vi "CheckAvailableFsample.vi"() -> ()   [LabVIEW 2022 SP3]
uses:
  <vilib>/Analysis/1siggen.llb/Ramp Pattern by Delta.vi
  <vilib>/DAQmx/configure/timing.llb/DAQmx Timing (Sample Clock).vi
  <resource>/objmgr/daqmx.rc
  <vilib>/Analysis/NI_AALBase.lvlib
  <vilib>/DAQmx/create/channels.llb/DAQmx Create Channel (AI-Voltage-Basic).vi
panel:
  out "error out":errorcluster
  in  "deltaFreq":dbl=1.0 format="%_3pHz"
  in  "minFreq":dbl=1.0 format="%_3pHz"
  in  "maxFreq":dbl=3000.0 format="%_3pHz"
  out "Fcheck":dbl
  out "XY Graph":cluster{dbl[], dbl[]}[](graph)
  in  "physical channels":tag
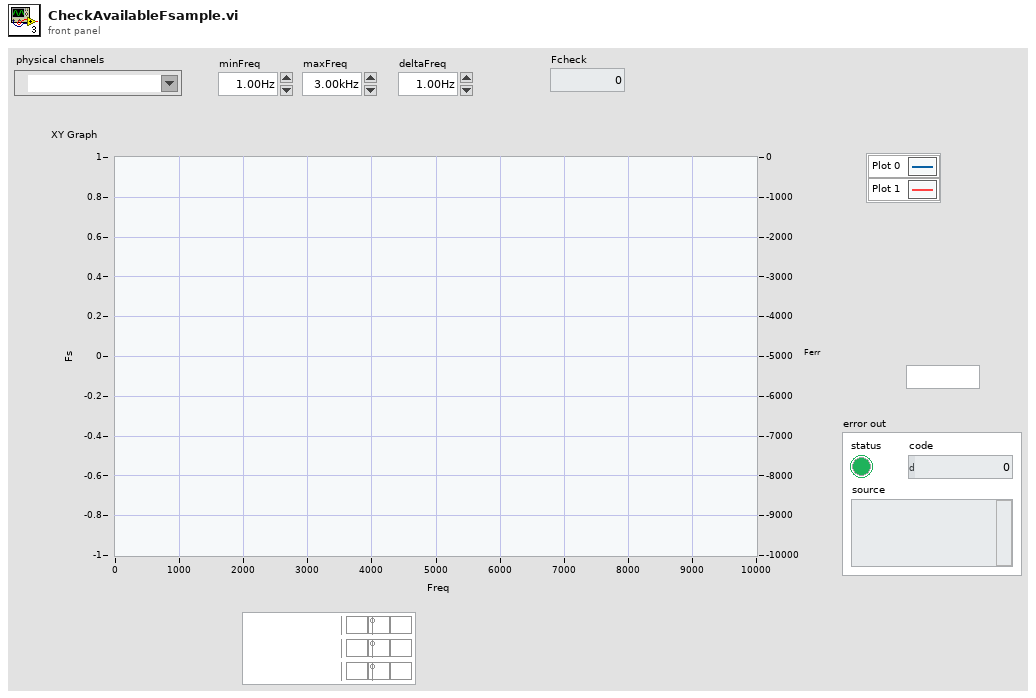
[diagram p1: front panel]
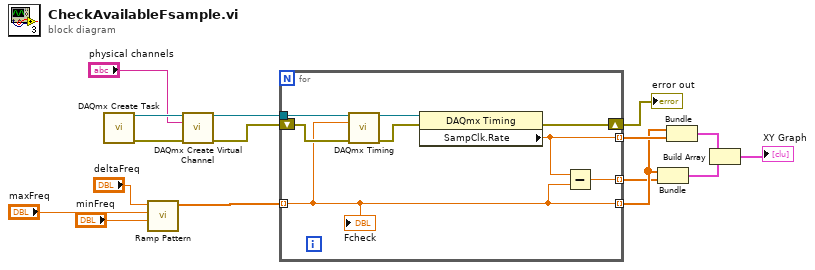
[diagram p0: block diagram]
diagram:
  n1 = call <vilib>:"DAQmx Create Task.vi"() -> ("task out"=w14:refnum<k21>, "error out"=w15:errorcluster)  [unwired: 14 in]
  n2 = call-poly <vilib>:"Ramp Pattern.vi"("start"="minFreq", "end"="maxFreq", "delta"="deltaFreq") -> ("Ramp Pattern"=w8:dbl[])  [unwired: 6 in, 2 out]
  n3 = call-poly <vilib>:"DAQmx Create Virtual Channel.vi"("task in"=w14, "physical channels"="physical channels", "error in"=w15) -> ("task out"=w13:refnum<k21>, "error out"=w16:errorcluster)  [unwired: 11 in]
  n4 = for {
    tunnel: w13 -> [w21]
    tunnel: w8 -> [w20] mode=indexing
    tunnel: [w19] -> w7 mode=indexing
    tunnel: [w20] -> w6 mode=indexing
    tunnel: [w18] -> w5 mode=indexing
    shift-right: [w17] -> w1
    shift-left: w16 -> [w22]
    n5 = call-poly <vilib>:"DAQmx Timing.vi"("task/channels in"=w21, "rate"=w20, "error in"=w22) -> ("task out"=w24:refnum<k21>, "error out"=w23:errorcluster)  [unwired: 4 in, 7 out]
    n6 = property class="DAQmx Timing"(reference=w24, error in=w23) -> (error out=w17:errorcluster, "SampClk.Rate"=w19:dbl)  [unwired: 1 out]
    n7 = Subtract(x=w19, y=w20) -> (x-y=w18:dbl)
    "Fcheck" <- w20
  }
  "error out" <- w1
  n8 = Bundle(w6, w5) -> (w3:cluster{dbl[], dbl[]})  [unwired: 1 in]
  n9 = Bundle(w6, w7) -> (w4:cluster{dbl[], dbl[]})  [unwired: 1 in]
  n10 = Build Array(w4, w3) -> (→"XY Graph":cluster{dbl[], dbl[]}[])
